vi "EventLogger-Init.vi"(7 "Device reference":refnum<vi>, 8 "error in (no error)":errorcluster, 10 "OutputRequest event ref":T1, 11 "InputData reference":refnum<vi>) -> (0 "error out":errorcluster, 2 "OutputRequest (dup)":T1, 3 "InputData (dup)":refnum<vi>)   [LabVIEW 2015]
doc: "Initializes an EventLogger device."
uses:
  Typedefs/EventLogger.ctl
  Rack/Typedefs/OutputRequest refnum.ctl
  Rack/Typedefs/OutputRequest.ctl
  Rack/Typedefs/InputData cluster.ctl
  Rack/Methods/Port drivers/DigitalInput-DataCluster.ctl
panel:
  # "Timestamp"
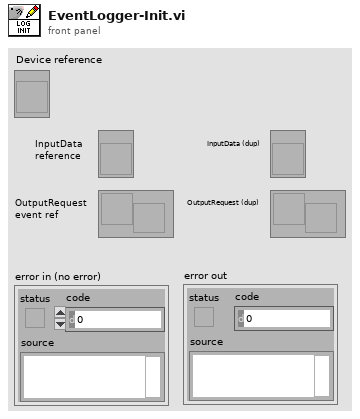
[diagram p1: front panel]
types:
  T1 = typedef "OutputRequest refnum.ctl" = refnum<user-event>
  T2 = typedef "EventLogger.ctl" = cluster{"Settings":cluster{"Portname":string, "Index":i32}, "OutputRequest event ref":T1, "InputData reference":refnum<vi>}
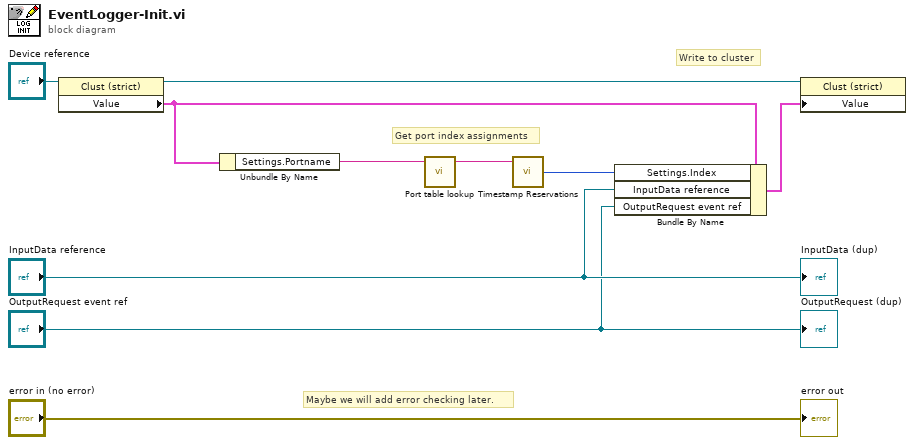
[diagram p0: block diagram]
diagram:
  # "Maybe we will add error checking later."
  # "Write to cluster"
  # "Get port index assignments"
  n1 = property class="Clust (strict)"(reference="Device reference") -> (reference out=w9:refnum<vi>, "Value"=w6:T2)  [unwired: 1 in, 1 out]
  n2 = Unbundle By Name(w6) -> ("Settings.Portname"=w4:string)
  n3 = call "Port table lookup.vi"("Port name"=w4) -> ("Line"=w7:tag)  [unwired: 3 in, 1 out]
  n4 = call "Timestamp Reservations.vi"("Line"=w7) -> ("Index assigned"=w5:i32)  [unwired: 2 in, 2 out]
  n5 = Bundle By Name(cluster=w6, "Settings.Index"=w5, "InputData reference"="InputData reference", "OutputRequest event ref"="OutputRequest event ref") -> (w8:T2)
  n6 = property class="Clust (strict)"(reference=w9, "Value"=w8) -> ()  [unwired: 1 in, 2 out]
  "error out" <- "error in (no error)"
  "OutputRequest (dup)" <- "OutputRequest event ref"
  "InputData (dup)" <- "InputData reference"
